vi "Global.vi"() -> ()   [LabVIEW 2020, in "GPP.lvlib"]
uses:
  GPP.lvlib
panel:
  out "Sys. History":cluster{"Boolean":bool}
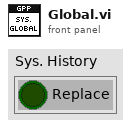
[diagram p1: front panel]
diagram:
